vi "datasourceConfigs.get.vi"(8 "error in (no error)":errorcluster, 11 "type in":refnum<class "type.lvclass">) -> (0 "error out":errorcluster, 2 "datasourceConfigs":T1[](array[typedef]), 3 "type out":refnum<class "type.lvclass">)   [LabVIEW 2020, in "type.lvclass"]
uses:
  type.lvclass
  datasourceConfig.ctl
  type.lvclass/type.ctl
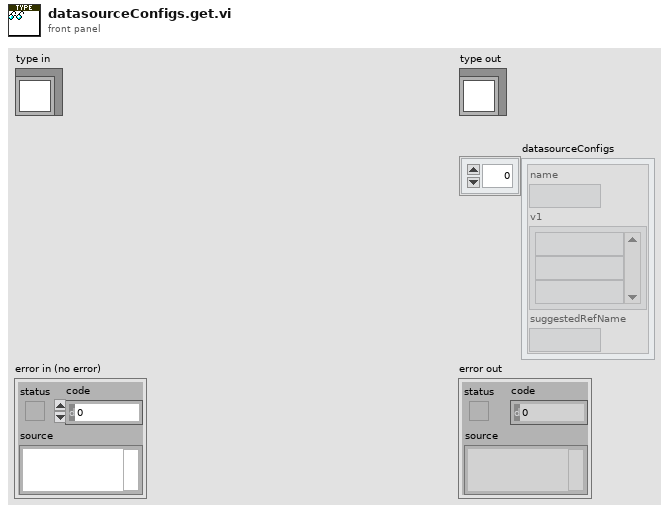
[diagram p1: front panel]
types:
  T1 = typedef "type.lvclass/datasourceConfig.ctl" = cluster{"name":string, "v1":string[], "suggestedRefName":string}
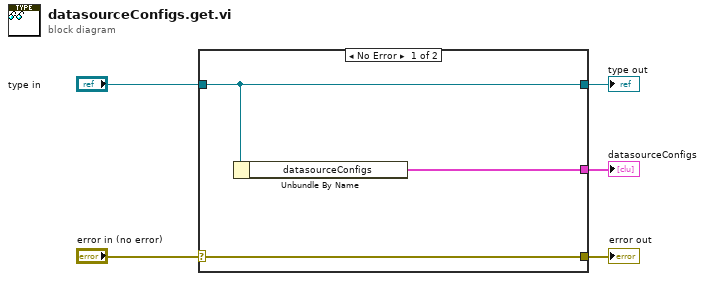
[diagram p0: block diagram]
diagram:
  n1 = case shown="No Error" "error in (no error)" {
    selector: "error in (no error)" -> [w8 w9]
    tunnel: [w8 w9] -> w4
    tunnel: [w7 w10] -> w2
    tunnel: "type in" -> [w7 w10]
    tunnel: [w6 _] -> w1
    frame No Error {
      n2 = Unbundle By Name(w7) -> ("datasourceConfigs"=w6:T1[])
    }
    frame Error {
    }
  }
  "error out" <- w4
  "type out" <- w2
  "datasourceConfigs" <- w1
